vi "Format Path into Python String.vi"(11 "Path":path) -> (3 "String":string)   [LabVIEW 2013, in "TS.lvlib"]
doc: "This VI formats the path to the Python script to be run so as to make it the first element of the Data array/list. Python will parse this on the other end, treating it like a relative path for platform-independence."
uses:
  TS.lvlib
panel:
  out "array of strings":string[](array[string])
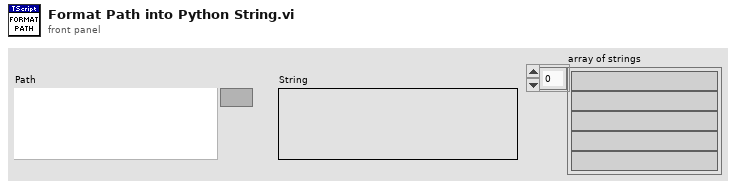
[diagram p1: front panel]
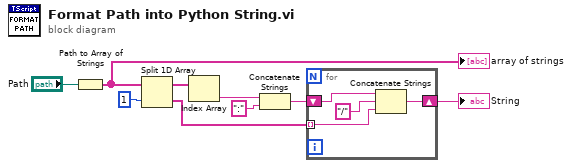
[diagram p0: block diagram]
diagram:
  n1 = Path to Array of Strings(0:"Path") -> (2:w6:string[])  [unwired: 1 out]
  "array of strings" <- w6
  n2 = Split 1D Array(array=w6, index=1) -> (first subarray=w5:string[], second subarray=w2:string[])
  n3 = Index Array(array=w5) -> (element=w4:string)  [unwired: 1 in]
  n4 = Concatenate Strings(w4, ":" ("string")) -> (w3:string)
  n5 = for {
    shift-right: [w13] -> w1
    shift-left: w3 -> [w12]
    tunnel: w2 -> [w10] mode=indexing
    n6 = Concatenate Strings(w12, "/" ("string"), w10) -> (w13:string)
  }
  "String" <- w1
